vi "Convert String to Engine.vi"(6 "initialize (first call)":bool, 7 "transfer group id":i32, 8 "error in":errorcluster, 9 "string buffer":refnum<class "Buffer.lvclass">, 10 "engine buffer":refnum<class "Buffer.lvclass">, 11 "DSF buffer converter in":refnum<class "Default Buffer Converter.lvclass">) -> (0 "error out":errorcluster, 3 "DSF buffer converter out":refnum<class "Default Buffer Converter.lvclass">)   [LabVIEW 2020, in "DSF Core.lvlib" / "Default Buffer Converter.lvclass"]
uses:
  Default Buffer Converter.lvclass
  Classes/Buffer/Buffer.lvclass
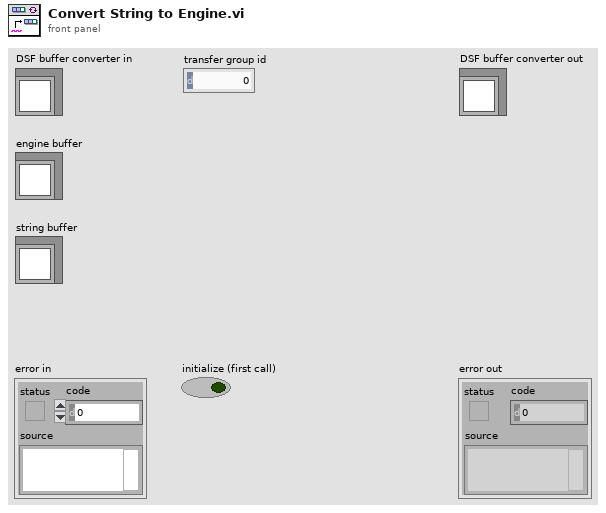
[diagram p1: front panel]
types:
  T1 = typedef "DSF Core.lvlib/Default Buffer Converter.lvclass/Conversion.ctl" = cluster{"conversion blocks":T2[]}
  T2 = typedef "DSF Core.lvlib/Default Buffer Converter.lvclass/Conversion Block.ctl" = cluster{"engine offset":u64, "engine data type":T3, "string offset":u64, "string data type":T3, "engine byte order":enum16{"big-endian, network order", "native, host order", "little-endian"}, "string byte order":enum16{"big-endian, network order", "native, host order", "little-endian"}, "count":u64}
  T3 = typedef "DSF Core.lvlib/DSF Data Type.ctl" = enum8{"Bool", "SGL", "DBL", "I8", "I16", "I32", "I64", "U8", "U16", "U32", "U64"}
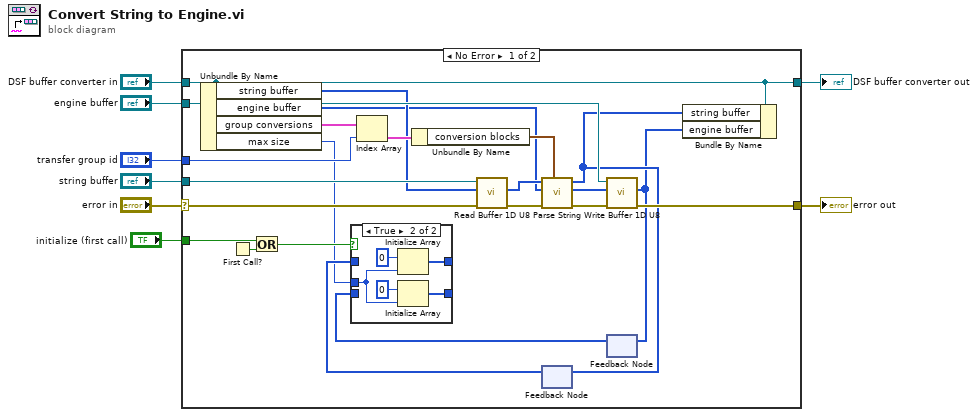
[diagram p0: block diagram]
diagram:
  n1 = case shown="No Error" "error in" {
    selector: "error in" -> [w20 w40]
    tunnel: [w19 w40] -> w7
    tunnel: [w12 w39] -> w5
    tunnel: "DSF buffer converter in" -> [w12 w39]
    tunnel: "transfer group id" -> [w29 _]
    tunnel: "string buffer" -> [w25 _]
    tunnel: "engine buffer" -> [w24 _]
    tunnel: "initialize (first call)" -> [w17 _]
    frame No Error {
      n2 = Unbundle By Name(w12) -> ("string buffer"=w13:u8[], "engine buffer"=w9:u8[], "group conversions"=w31:T1[], "max size"=w14:u64)
      n3 = First Call?() -> (First Call?: T/F=w16:bool)
      n4 = Or(x=w17, y=w16) -> (x .or. y?=w15:bool)
      n5 = Index Array(array=w31, index=w29) -> (element=w30:T1)
      n6 = Unbundle By Name(w30) -> ("conversion blocks"=w18:T2[])
      n7 = call "Read Buffer 1D U8.vi"("error in (no error)"=w20, "dst array in"=w13, "Buffer in"=w25) -> ("error out"=w28:errorcluster, "dst array out"=w26:u8[])  [unwired: 5 in, 2 out]
      n8 = call "Parse String.vi"("conversion blocks"=w18, "error in (no error)"=w28, "engine buffer in"=w9, "string buffer in"=w26) -> ("error out"=w27:errorcluster, "engine buffer out"=w23:u8[], "string buffer out"=w11:u8[])  [unwired: 5 in]
      n9 = feedback #1() -> (w22:u8[])  [unwired: 1 in]
      n10 = feedback-in #1(w11) -> ()
      n11 = call "Write Buffer 1D U8.vi"("error in (no error)"=w27, "src array in"=w23, "Buffer in"=w24) -> ("error out"=w19:errorcluster, "src array out"=w10:u8[])  [unwired: 5 in, 2 out]
      n12 = feedback #2() -> (w21:u8[])  [unwired: 1 in]
      n13 = case shown="True" w15 {
        tunnel: w14 -> [_ w34]
        tunnel: [w32 w37] -> _
        tunnel: [w33 w35] -> _
        tunnel: w21 -> [w33 _]
        tunnel: w22 -> [w32 _]
        frame False {
        }
        frame True {
          n14 = Initialize Array(u8 0 ("element"), w34) -> (w37:u8[])
          n15 = Initialize Array(u8 0 ("element"), w34) -> (w35:u8[])
        }
      }
      n16 = feedback-in #2(w10) -> ()
      n17 = Bundle By Name(cluster=w12, "string buffer"=w11, "engine buffer"=w10) -> ()  [unwired: 1 out]
    }
    frame Error {
    }
  }
  "error out" <- w7
  "DSF buffer converter out" <- w5
